vi "Save Data.vi"(8 "error in (no error)":errorcluster, 9 "Data":bool[](array[boolean]), 11 "Digital Acquisition in":refnum<class "Digital Acquisition.lvclass">) -> (0 "error out":errorcluster, 3 "Digital Acquisition out":refnum<class "Digital Acquisition.lvclass">)   [LabVIEW 2020, in "Digital Acquisition.lvlib" / "Digital Acquisition.lvclass"]
uses:
  Digital Acquisition.lvclass
  Digital Acquisition.lvclass/Digital Acquisition.ctl
  Digital Logging/Digital Logging Messages/Save Digital Data Msg/Save Digital Data Msg.lvclass/Save Digital Data Msg.ctl
  <vilib>/ActorFramework/Message Enqueuer/Message Enqueuer.lvclass/Message Enqueuer.ctl
  <vilib>/ActorFramework/Message Enqueuer/Enqueue.vi
  Digital Logging/Digital Logging Messages/Save Digital Data Msg/Save Digital Data Msg.lvclass
  C:/Program Files (x86)/National Instruments/LabVIEW 2020/vi.lib/ActorFramework/Message/Message.lvclass
  <vilib>/ActorFramework/Message Priority Queue/Priority Enqueue.vi
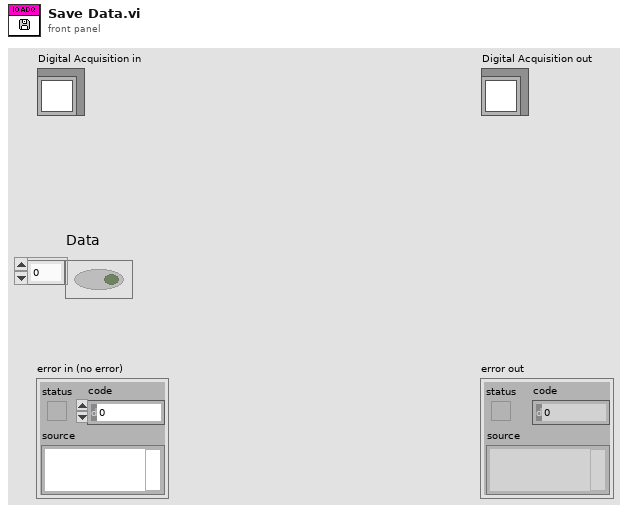
[diagram p1: front panel]
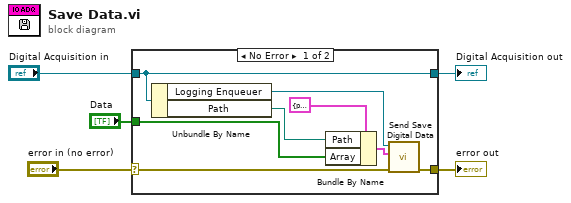
[diagram p0: block diagram]
diagram:
  n1 = case shown="No Error" "error in (no error)" {
    selector: "error in (no error)" -> [w11 w15]
    tunnel: [w10 w15] -> w4
    tunnel: [w13 w14] -> w2
    tunnel: "Digital Acquisition in" -> [w13 w14]
    tunnel: "Data" -> [w8 _]
    frame No Error {
      n2 = Unbundle By Name(w13) -> ("Logging Enqueuer"=w12:refnum<class "Message Enqueuer.lvclass">, "Path"=w6:path)
      n3 = Bundle By Name(cluster=cluster{"Path":path, "Array":bool[]} {"Path"=path "", "Array"=[]} ("Data Cluster"), "Path"=w6, "Array"=w8) -> (w7:cluster{"Path":path, "Array":bool[]})
      n4 = call "Send Save Digital Data.vi"("error in (no error)"=w11, "Data Cluster"=w7, "Message Enqueuer"=w12) -> ("error out"=w10:errorcluster)  [unwired: 7 in, 1 out]
    }
    frame Error {
    }
  }
  "error out" <- w4
  "Digital Acquisition out" <- w2
